vi "SO2 calc PID.vi"(4 "I":dbl, 6 "Feed":dbl, 7 "P":dbl, 8 "Flow Rate":dbl, 9 "SO2 Measured ppm":dbl, 10 "SO2 Conc":dbl, 11 "SO2 Target ppm":dbl) -> (2 "SO2 MFR":dbl)   [LabVIEW 2011]
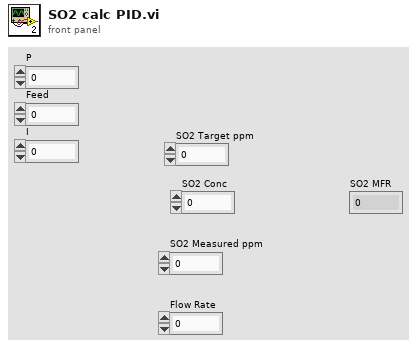
[diagram p1: front panel]
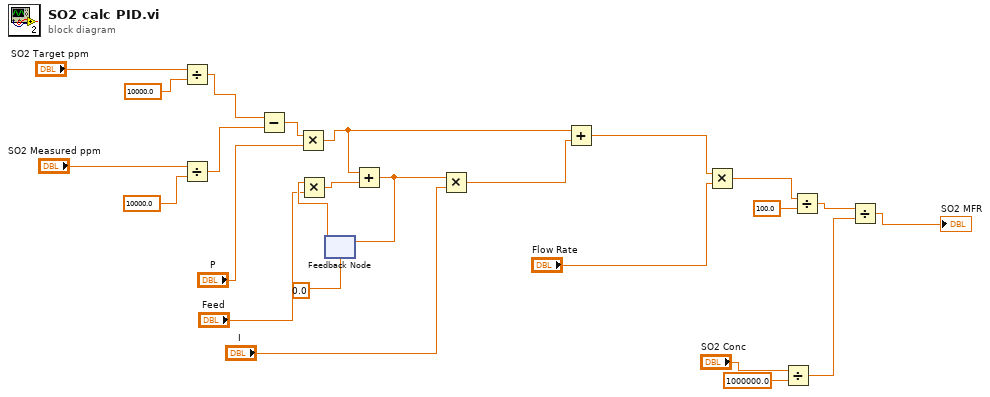
[diagram p0: block diagram]
diagram:
  n1 = Divide(x="SO2 Target ppm", y=10000.0) -> (x/y=w14:dbl)
  n2 = Divide(x="SO2 Measured ppm", y=10000.0) -> (x/y=w15:dbl)
  n3 = Subtract(x=w14, y=w15) -> (x-y=w13:dbl)
  n4 = Multiply(x=w13, y="P") -> (x*y=w11:dbl)
  n5 = feedback #1(0.0) -> (w6:dbl)
  n6 = Multiply(x=w6, y="Feed") -> (x*y=w5:dbl)
  n7 = Add(x=w11, y=w5) -> (x+y=w7:dbl)
  n8 = feedback-in #1(w7) -> ()
  n9 = Multiply(x=w7, y="I") -> (x*y=w10:dbl)
  n10 = Add(x=w11, y=w10) -> (x+y=w9:dbl)
  n11 = Multiply(x=w9, y="Flow Rate") -> (x*y=w20:dbl)
  n12 = Divide(x="SO2 Conc", y=1000000.0) -> (x/y=w16:dbl)
  n13 = Divide(x=w20, y=100.0) -> (x/y=w19:dbl)
  n14 = Divide(x=w19, y=w16) -> (x/y=→"SO2 MFR":dbl)
